vi "Take histogram.vi"() -> ()   [LabVIEW 2017, in "GP22_TDC_Arduinoed.lvlib"]
uses:
  GP22_TDC_Arduinoed.lvlib
panel:
  in  "Histogram minimum / ns (0)":dbl
  in  "Histogram maximum / ns (100)":dbl=100.0
  in  "# bins":i32=100
  in  "Time in ms (30000)":u32=5000
  out "Timing histogram":T1(graph)
  out "error out":errorcluster
  in  "VISA resource name":refnum<visa-resource-name>
  # "This VI asks the TDC to create a histogram\nof results between two times. \n\nThis method is quick compared to the\n\"multiple measurements\" command, however the user must set the bounds themselves and any measurements which fall outside those bounds will be missed."
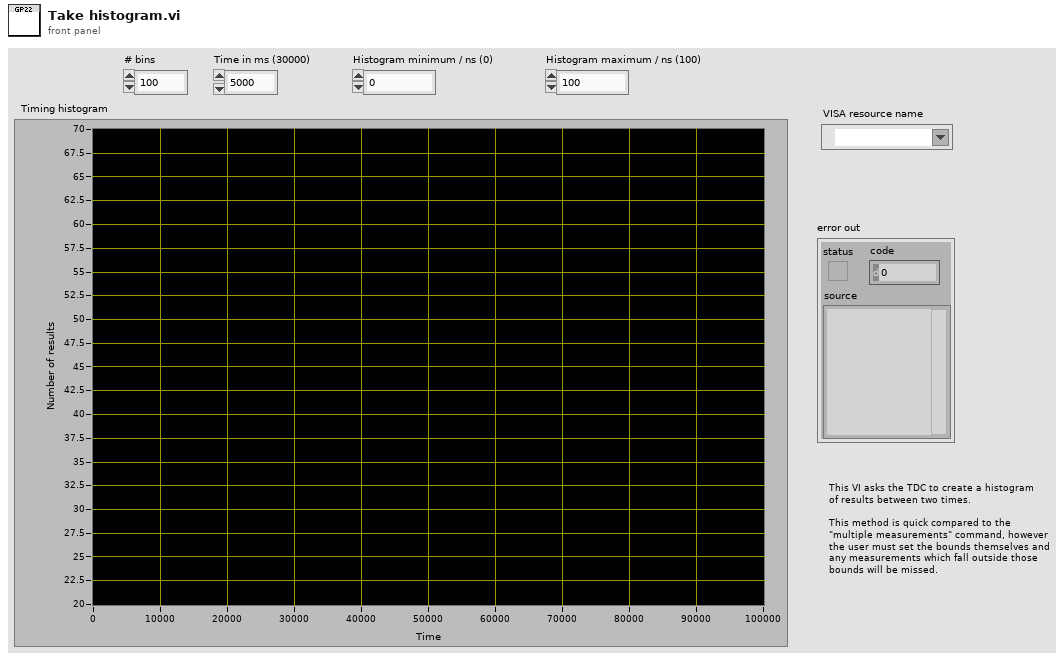
[diagram p1: front panel]
types:
  T1 = cluster{"Unbinned times / s":dbl[], "Binned time":dbl[]}
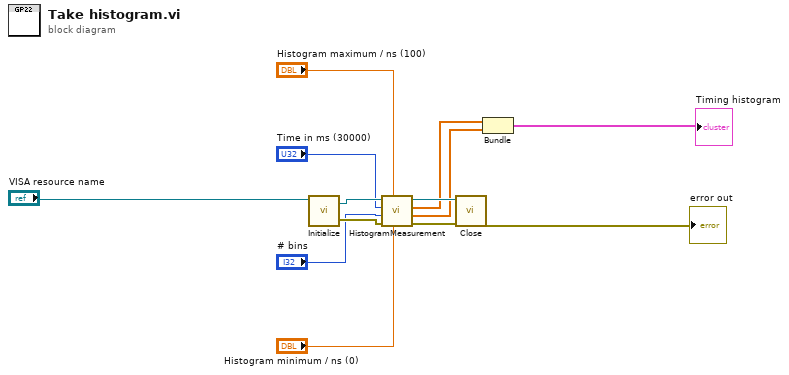
[diagram p0: block diagram]
diagram:
  n1 = call "Initialize.vi"("VISA resource name"="VISA resource name") -> ("error out"=w10:errorcluster, "VISA resource name out"=w13:refnum<visa-resource-name>)  [unwired: 5 in]
  n2 = call "HistogramMeasurement.vi"("Histogram minimum / ns (0)"="Histogram minimum / ns (0)", "Histogram maximum / ns (100)"="Histogram maximum / ns (100)", "error in (no error)"=w10, "Number of bins (50)"="# bins", "Time to measure (1000)"="Time in ms (30000)", "VISA resource name"=w13) -> ("error out"=w9:errorcluster, "Counts"=w3:dbl[], "Times / ns"=w4:dbl[], "VISA resource name out"=w12:refnum<visa-resource-name>)  [unwired: 2 in]
  n3 = call "Close.vi"("error in (no error)"=w9, "VISA resource name"=w12) -> ("error out"=→"error out":errorcluster)  [unwired: 9 in]
  n4 = Bundle("Times / ns"=w4, "Counts"=w3) -> (→"Timing histogram":cluster{"Times / ns":dbl[], "Counts":dbl[]})  [unwired: 1 in]
